vi "PPMS2_Log_Parse.vi"(11 "file path (dialog if empty)":path=path "C:/Users/Pittsburgh/Desktop/PPMS2 Log/ppms2log_201604120.dat") -> (2 "XY Graph":cluster{timestamp[], dbl[]}[](graph), 3 "Array":string[](array[string])=["PPMS2 Comment", "PPMS2 Time Stamp (sec)", "PPMS2 Status (code)", "PPMS2 Temperature (K)", "PPMS2 Magnetic Field (Oe)", "PPMS2 Sample Position (deg)", "PPMS2 Bridge 1 Resistance (ohms)", "PPMS2 Bridge 1 Excitation (uA)", "PPMS2 Bridge 2 Resistance (ohms)", "PPMS2 Bridge 2 Excitation (uA)", "PPMS2 Bridge 3 Resistance (ohms)", "PPMS2 Bridge 3 Excitation (uA)", "PPMS2 Bridge 4 Resistance (ohms)", "PPMS2 Bridge 4 Excitation (uA)", "PPMS2 Signal 1 Vin (V)", "PPMS2 Signal 2 Vin (V)", "PPMS2 Digital Inputs (code)", "PPMS2 Drive 1 Iout (mA)", "PPMS2 Drive 1 Ipower (watts)", "PPMS2 Drive 2 Iout (mA)", "PPMS2 Drive 2 Ipower (watts)", "PPMS2 Pressure ()", "PPMS2 Map 20 ()", "PPMS2 Map 21 ()", "PPMS2 Map 22 ()", "PPMS2 Map 23 ()", "PPMS2 Map 24 ()", "PPMS2 Map 25 ()", "PPMS2 Map 26 ()", "PPMS2 Map 27 ()", "PPMS2 Map 28 ()", "PPMS2 Map 29 ()", "PPMS2 System Status (code)", "PPMS2 Setpoint (K)", "PPMS2 Magnet (Oe)", "PPMS2 Valve Position (deg)", "PPMS2 CIG Cernox (K)", "PPMS2 CIG Excit (uA)", "PPMS2 Plat Therm (K)", "PPMS2 Plat Excit (uA)", "PPMS2 Neck Therm (K)", "PPMS2 Neck Excit (uA)", "PPMS2 Spare Therm (K)", "PPMS2 Spare Excit (uA)", "PPMS2 Flow Rate (l min)", "PPMS2 Annulus Vacuum (V)", "PPMS2 Impedance (mode)", "PPMS2 Block Htr Cur (mA)", "PPMS2 Block Htr Pwr (W)", "PPMS2 Neck Htr Cur (mA)", "PPMS2 Neck Htr Pwr (W)", "PPMS2 Annulus Pres (Torr)", "PPMS2 System Pres (Torr)", "PPMS2 Tableless Map53 ()", "PPMS2 Tableless Map54 ()", "PPMS2 Redirected 55 ()", "PPMS2 Redirected 56 ()", "PPMS2 Redirected 57 ()", "PPMS2 Redirected 58 ()", "PPMS2 Redirected 59 ()", "PPMS2 EXT Flow (L min)", "PPMS2 Redirected 61 ()", "PPMS2 Seq Stat ()", "PPMS2 Sys Temp ()", "PPMS2 He Level ()", "PPMS2 Map 67 ()", "PPMS2 Map 68 ()", "PPMS2 Map 69 ()", "PPMS2 PSU Field (Oe)", "PPMS2 Hi res (A) read", "PPMS2 Mag (V) read", "PPMS2 Mag adj sc(I)set", "PPMS2 Sw heater state", "PPMS2 DAC  I  (cnts)", "PPMS2 Therm v", "PPMS2 KRPMs", "PPMS2 Pump temp (C)", "PPMS2 Pump power (W)", "PPMS2 High Vacuum mode", "PPMS2 Flapper state", "PPMS2 Regen htr flag", "PPMS2 iso flag", "PPMS2 BlockHeater(Ohm)", "PPMS2 NeckHeater(Ohm)", "PPMS2 Last 2 eng st", "PPMS2 Hires enable", "PPMS2 Mag (V) set", "PPMS2 Map 89 ()", "PPMS2 Map 90 ()", "PPMS2 Map 91 ()", "PPMS2 Map 92 ()", "PPMS2 Map 93 ()"])   [LabVIEW 2013]
uses:
  <vilib>/Utility/file.llb/Read From Spreadsheet File (string).vi
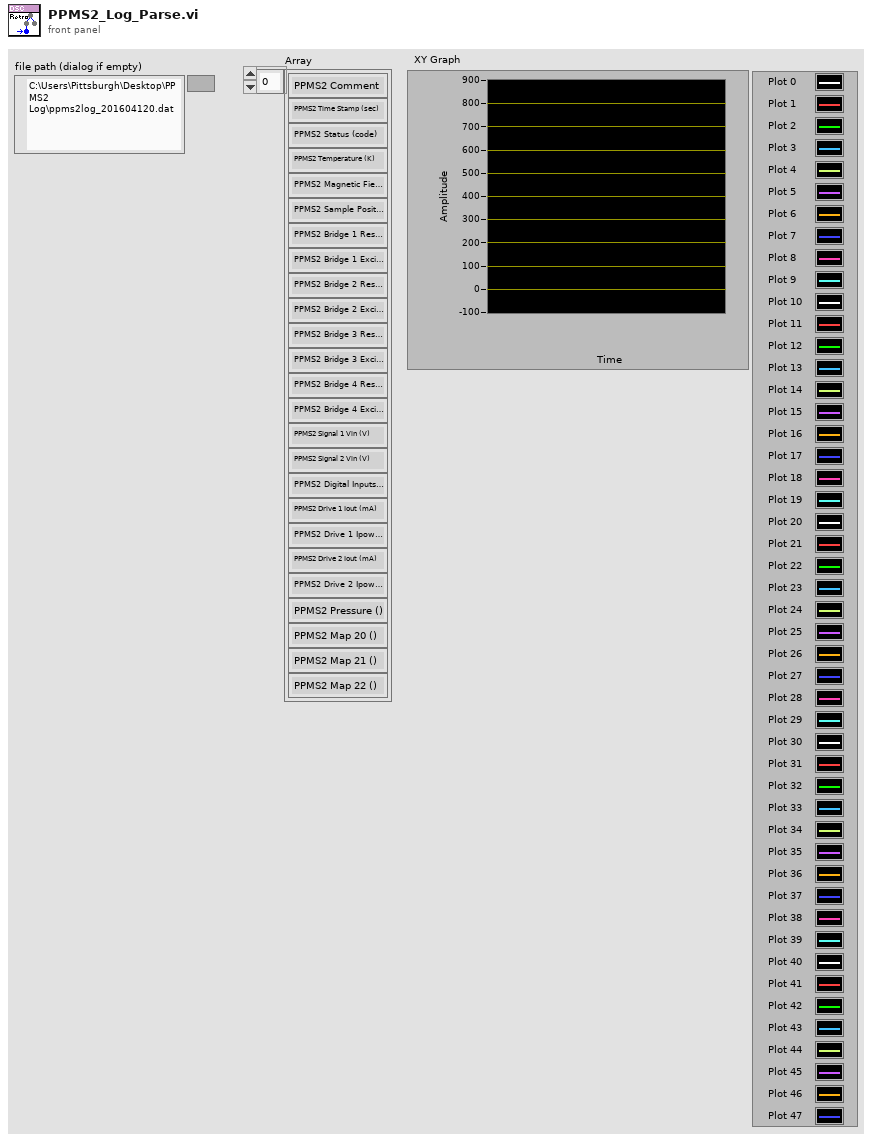
[diagram p1: front panel]
types:
  T1 = cluster{"second":i32, "minute":i32, "hour":i32, "day of month":i32, "month":i32, "year":i32, "day of week":i32, "day of year":i32, "is DST":i32}
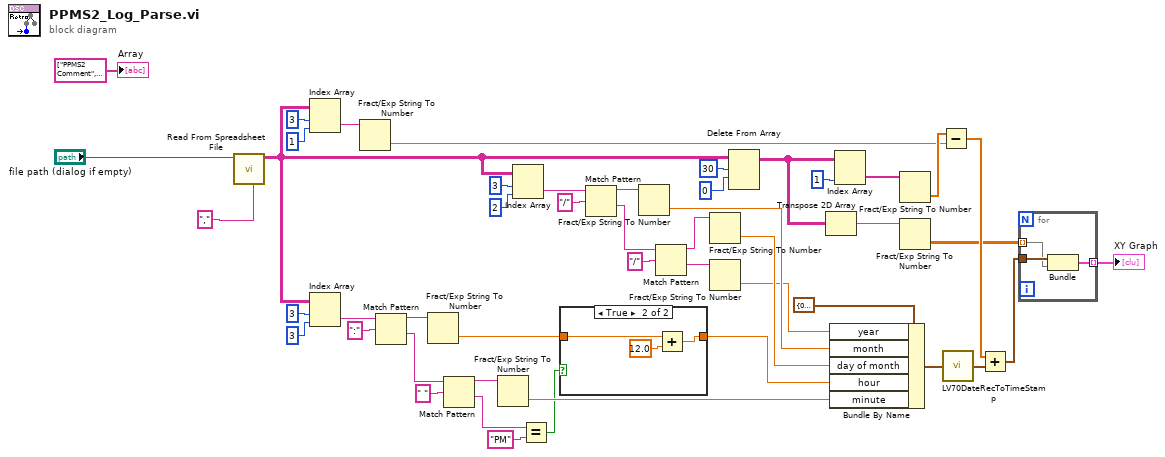
[diagram p0: block diagram]
diagram:
  n1 = call-poly <vilib>:"Read From Spreadsheet File.vi"("delimiter (\\t)"="," ("delimiter (\\t)"), "file path (dialog if empty)"="file path (dialog if empty)") -> ("all rows"=w8:string[][])  [unwired: 5 in, 4 out]
  n2 = Index Array(array=w8, index (row)=3, index (col)=1 ("disabled index (col)")) -> (element=w13:string)
  n3 = Index Array(array=w8, index (row)=3, index (col)=3 ("disabled index (col)")) -> (element=w26:string)
  n4 = Fract/Exp String To Number(string=w13) -> (number=w11:dbl)  [unwired: 3 in, 1 out]
  n5 = Match Pattern(string=w26, regular expression=":" ("search string/char (-)")) -> (before substring=w25:string, after substring=w24:string)  [unwired: 1 in, 2 out]
  n6 = Fract/Exp String To Number(string=w25) -> (number=w17:dbl)  [unwired: 3 in, 1 out]
  n7 = Match Pattern(string=w24, regular expression=" ") -> (before substring=w22:string, after substring=w20:string)  [unwired: 1 in, 2 out]
  n8 = Fract/Exp String To Number(string=w22) -> (number=w21:dbl)  [unwired: 3 in, 1 out]
  n9 = Index Array(array=w8, index (row)=3, index (col)=2 ("disabled index (col)")) -> (element=w39:string)
  n10 = Equal?(x=w20, y="PM") -> (x = y?=w18:bool)
  n11 = case shown="True" w18 {
    tunnel: w17 -> [w49 w52]
    tunnel: [w49 w50] -> w16
    frame False {
    }
    frame True {
      n12 = Add(x=w52, y=12.0) -> (x+y=w50:dbl)
    }
  }
  n13 = Match Pattern(string=w39, regular expression="/" ("search string/char (-)")) -> (before substring=w34:string, after substring=w29:string)  [unwired: 1 in, 2 out]
  n14 = Fract/Exp String To Number(string=w34) -> (number=w33:dbl)  [unwired: 3 in, 1 out]
  n15 = Match Pattern(string=w29, regular expression="/" ("search string/char (-)")) -> (before substring=w32:string, after substring=w28:string)  [unwired: 1 in, 2 out]
  n16 = Fract/Exp String To Number(string=w32) -> (number=w31:dbl)  [unwired: 3 in, 1 out]
  n17 = Fract/Exp String To Number(string=w28) -> (number=w30:dbl)  [unwired: 3 in, 1 out]
  n18 = Delete From Array(array=w8, length=30, index (row)=0) -> (array with subset deleted=w7:string[][])  [unwired: 1 in, 1 out]
  n19 = Transpose 2D Array(2D array=w7) -> (transposed array=w6:string[][])
  n20 = Bundle By Name(cluster=T1 {"second"=0, "minute"=0, "hour"=0, "day of month"=0, "month"=0, "year"=0, "day of week"=0, "day of year"=0, "is DST"=0} ("date time rec"), "year"=w30, "month"=w33, "day of month"=w31, "hour"=w16, "minute"=w21) -> (w36:T1)
  n21 = Index Array(array=w7, index (col)=1 ("disabled index (col)")) -> (element=w46:string[])  [unwired: 1 in]
  n22 = Fract/Exp String To Number(string=w46) -> (number=w12:dbl[])  [unwired: 3 in, 1 out]
  n23 = Fract/Exp String To Number(string=w6) -> (number=w4:dbl[][])  [unwired: 3 in, 1 out]
  n24 = Subtract(x=w12, y=w11) -> (x-y=w9:dbl[])
  n25 = call <vilib>:"LV70DateRecToTimeStamp.vi"("date time rec"=w36) -> ("Time Stamp"=w10:timestamp)
  n26 = Add(x=w9, y=w10) -> (x+y=w5:timestamp[])
  n27 = for {
    tunnel: w5 -> [w55]
    tunnel: w4 -> [w54] mode=indexing
    tunnel: [w53] -> w2 mode=indexing
    n28 = Bundle(w55, w54) -> (w53:cluster{timestamp[], dbl[]})  [unwired: 1 in]
  }
  "XY Graph" <- w2
  "Array" <- string[] ["PPMS2 Comment", "PPMS2 Time Stamp (sec)", "PPMS2 Status (code)", "PPMS2 Temperature (K)", "PPMS2 Magnetic Field (Oe)", "PPMS2 Sample Position (deg)", "PPMS2 Bridge 1 Resistance (ohms)", "PPMS2 Bridge 1 Excitation (uA)", "PPMS2 Bridge 2 Resistance (ohms)", "PPMS2 Bridge 2 Excitation (uA)", "PPMS2 Bridge 3 Resistance (ohms)", "PPMS2 Bridge 3 Excitation (uA)", "PPMS2 Bridge 4 Resistance (ohms)", "PPMS2 Bridge 4 Excitation (uA)", "PPMS2 Signal 1 Vin (V)", "PPMS2 Signal 2 Vin (V)", "PPMS2 Digital Inputs (code)", "PPMS2 Drive 1 Iout (mA)", "PPMS2 Drive 1 Ipower (watts)", "PPMS2 Drive 2 Iout (mA)", "PPMS2 Drive 2 Ipower (watts)", "PPMS2 Pressure ()", "PPMS2 Map 20 ()", "PPMS2 Map 21 ()", "PPMS2 Map 22 ()", "PPMS2 Map 23 ()", "PPMS2 Map 24 ()", "PPMS2 Map 25 ()", "PPMS2 Map 26 ()", "PPMS2 Map 27 ()", "PPMS2 Map 28 ()", "PPMS2 Map 29 ()", "PPMS2 System Status (code)", "PPMS2 Setpoint (K)", "PPMS2 Magnet (Oe)", "PPMS2 Valve Position (deg)", "PPMS2 CIG Cernox (K)", "PPMS2 CIG Excit (uA)", "PPMS2 Plat Therm (K)", "PPMS2 Plat Excit (uA)", "PPMS2 Neck Therm (K)", "PPMS2 Neck Excit (uA)", "PPMS2 Spare Therm (K)", "PPMS2 Spare Excit (uA)", "PPMS2 Flow Rate (l min)", "PPMS2 Annulus Vacuum (V)", "PPMS2 Impedance (mode)", "PPMS2 Block Htr Cur (mA)", "PPMS2 Block Htr Pwr (W)", "PPMS2 Neck Htr Cur (mA)", "PPMS2 Neck Htr Pwr (W)", "PPMS2 Annulus Pres (Torr)", "PPMS2 System Pres (Torr)", "PPMS2 Tableless Map53 ()", "PPMS2 Tableless Map54 ()", "PPMS2 Redirected 55 ()", "PPMS2 Redirected 56 ()", "PPMS2 Redirected 57 ()", "PPMS2 Redirected 58 ()", "PPMS2 Redirected 59 ()", "PPMS2 EXT Flow (L min)", "PPMS2 Redirected 61 ()", "PPMS2 Seq Stat ()", "PPMS2 Sys Temp ()", "PPMS2 He Level ()", "PPMS2 Map 67 ()", "PPMS2 Map 68 ()", "PPMS2 Map 69 ()", "PPMS2 PSU Field (Oe)", "PPMS2 Hi res (A) read", "PPMS2 Mag (V) read", "PPMS2 Mag adj sc(I)set", "PPMS2 Sw heater state", "PPMS2 DAC  I  (cnts)", "PPMS2 Therm v", "PPMS2 KRPMs", "PPMS2 Pump temp (C)", "PPMS2 Pump power (W)", "PPMS2 High Vacuum mode", "PPMS2 Flapper state", "PPMS2 Regen htr flag", "PPMS2 iso flag", "PPMS2 BlockHeater(Ohm)", "PPMS2 NeckHeater(Ohm)", "PPMS2 Last 2 eng st", "PPMS2 Hires enable", "PPMS2 Mag (V) set", "PPMS2 Map 89 ()", "PPMS2 Map 90 ()", "PPMS2 Map 91 ()", "PPMS2 Map 92 ()", "PPMS2 Map 93 ()"] ("Array 2")
